vi "Read Measurement (Time Voltage Interval).vi"(0 "VISA resource name":refnum<visa-resource-name>, 1 "Slope (0:Positive)":i32(ring) items=["Positive", "Negative"], 2 "Occurrence (3)":i32 format="%.0g", 5 "Channel (1: Channel 1)":u16(ring) items=["Channel 1", "Channel 2", "Channel 3", "Channel 4", "Function 1", "Function 2", "Function 3", "Function 4", "Memory 1", "Memory 2", "Memory 3", "Memory 4"], 7 "Voltage Level (-0.25)":dbl, 9 "Maximum Time (10000ms)":u32, 11 "error in (no error)":errorcluster) -> (4 "VISA resource name out":refnum<visa-resource-name>, 6 "Time Interval (s)":dbl, 15 "error out":errorcluster)   [LabVIEW 2009, in "Agilent 8000 Series.lvlib"]
doc: "Returns the voltage at a specified time. The specified time must be on screen and referenced to the trigger event.\n\nThis VI initiates an acquisition on the channel that the end-user defined. It then waits for the acquisition to complete, obtains a waveform measurement on the channel the end-user specifies, and returns the measurement value."
uses:
  Agilent 8000 Series.lvlib
  Low Level/Fetch Measurement (Time Voltage Interval).vi
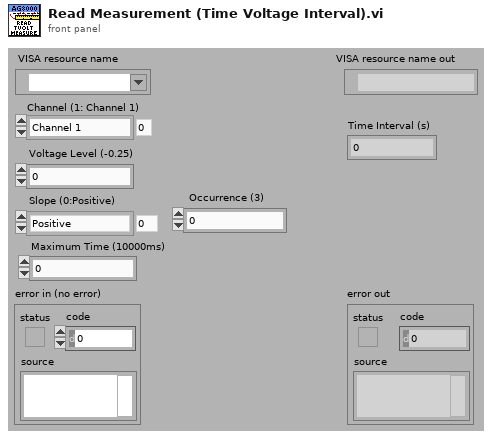
[diagram p1: front panel]
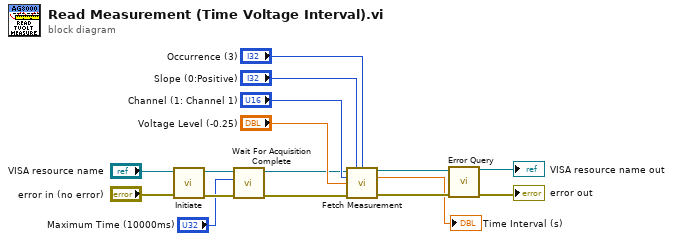
[diagram p0: block diagram]
diagram:
  n1 = call "Initiate.vi"("error in (no error)"="error in (no error)", "VISA resource name"="VISA resource name") -> ("error out"=w6:errorcluster, "VISA resource name out"=w7:refnum<visa-resource-name>)  [unwired: 8 in]
  n2 = call "Wait For Acquisition Complete.vi"("error in (no error)"=w6, "Maximum Time (10000ms)"="Maximum Time (10000ms)", "VISA resource name"=w7) -> ("error out"=w5:errorcluster, "VISA resource name out"=w4:refnum<visa-resource-name>)  [unwired: 7 in]
  n3 = call-poly "Fetch Measurement.vi"("VISA resource name"=w4, "Slope (0: Positive)"="Slope (0:Positive)", "Occurrence (3)"="Occurrence (3)", "Channel (1: Channel 1)"="Channel (1: Channel 1)", "Voltage Level (-0.25)"="Voltage Level (-0.25)", "error in (no error)"=w5) -> ("VISA resource name out"=w12:refnum<visa-resource-name>, "Time Interval (s)"=→"Time Interval (s)":dbl, "error out"=w11:errorcluster)  [unwired: 7 in]
  n4 = call "Error Query.vi"("error in (no error)"=w11, "VISA resource name"=w12) -> ("error out"=→"error out":errorcluster, "VISA resource name out"=→"VISA resource name out":refnum<visa-resource-name>)  [unwired: 6 in, 2 out]
